vi "Boolean Stop After X or When Released.vi"(1 "Min Time Pressed":u64=1000, 2 "Go":bool) -> (0 "Output":bool)   [LabVIEW 2015]
panel:
  out "millisecond timer value":u32
  in  "Time To Go":u32
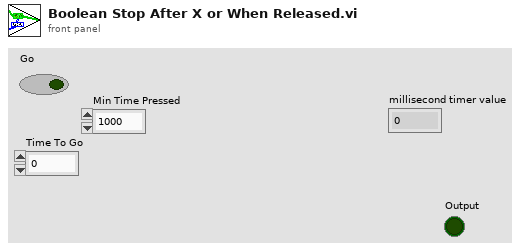
[diagram p1: front panel]
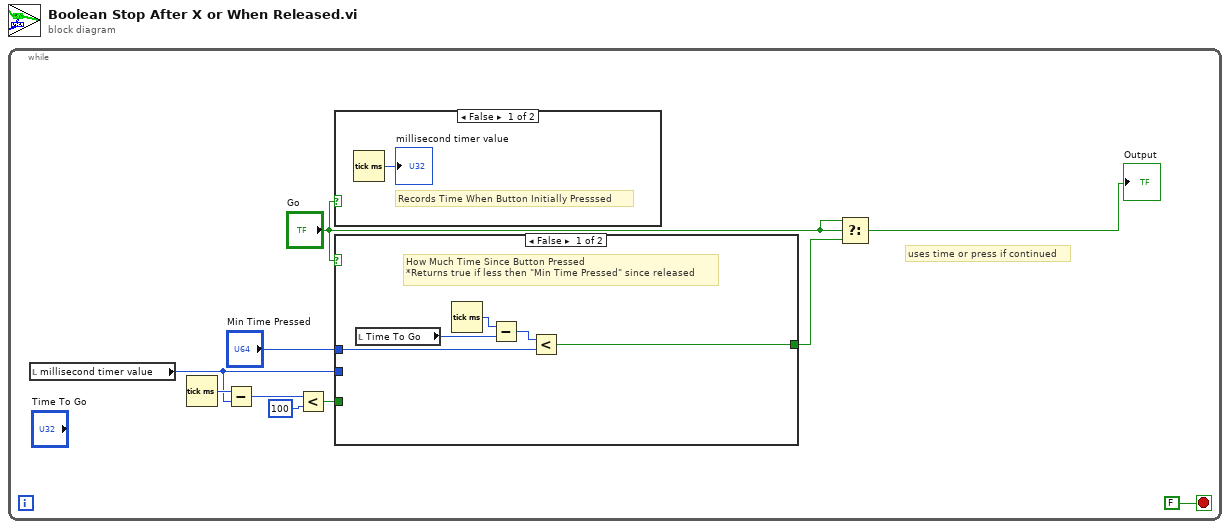
[diagram p0: block diagram]
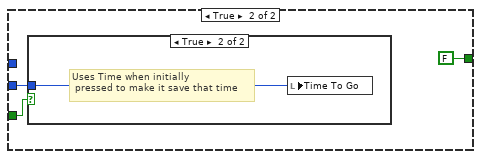
[diagram p3: hidden frame]
diagram:
  n1 = while {
    stop <- FALSE stop-if-true
    # "uses time or press if continued"
    n2 = local read "millisecond timer value"() -> (w4:u32)
    n3 = Tick Count (ms)() -> (millisecond timer value=w8:u32)
    n4 = Subtract(x=w8, y=w4) -> (x-y=w7:u32)
    n5 = Less?(x=w7, y=u32 100) -> (x < y?=w5:bool)
    n6 = case shown="False" "Go" {
      frame False {
        # "Records Time When Button Initially Presssed"
        n7 = Tick Count (ms)() -> (millisecond timer value=→"millisecond timer value":u32)
      }
      frame True {
      }
    }
    n8 = case shown="False" "Go" {
      tunnel: "Min Time Pressed" -> [w13 _]
      tunnel: [w12 FALSE] -> w9
      tunnel: w5 -> [_ w18]
      tunnel: w4 -> [_ w17]
      frame False {
        # "How Much Time Since Button Pressed\n*Returns true if less then \"Min Time Pressed\" since released"
        n9 = local read "Time To Go"() -> (w15:u32)
        n10 = Tick Count (ms)() -> (millisecond timer value=w14:u32)
        n11 = Subtract(x=w14, y=w15) -> (x-y=w16:u32)
        n12 = Less?(x=w16, y=w13) -> (x < y?=w12:bool)
      }
      frame True {
        n13 = case shown="True" w18 {
          tunnel: w17 -> [_ w20]
          frame False {
          }
          frame True {
            # "Uses Time when initially\n pressed to make it save that time"
            n14 = local write "Time To Go"(w20) -> ()
          }
        }
      }
    }
    n15 = Select(t="Go", s="Go", f=w9) -> (s? t:f=→"Output":bool)
  }
